vi "inst.Open.vi"(7 "unit ID in":u8=11, 8 "error in (no error)":errorcluster, 11 "VISA resource name":refnum<visa-resource-name>="COM4") -> (0 "error out":errorcluster, 3 "Modbus Master out":refnum<class "Modbus Master.lvclass">)   [LabVIEW 2018, in "MB Relay.lvlib"]
uses:
  MB Relay.lvlib
  <vilib>/NI/Modbus Library/API/Master/Modbus Master.lvclass
  <vilib>/NI/Modbus Library/API/Wrapper/Create Serial Master.vi
  <vilib>/NI/Modbus Library/API/Wrapper/API Main.lvlib
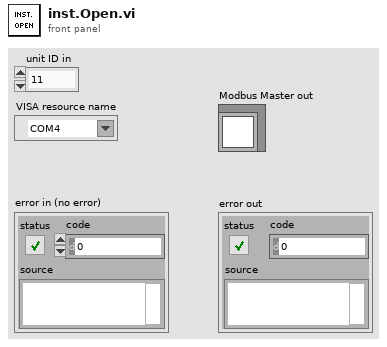
[diagram p1: front panel]
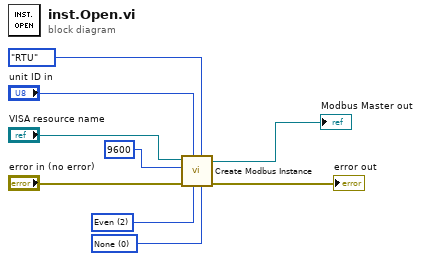
[diagram p0: block diagram]
diagram:
  w6 = u16 0 items=["None", "XON/XOFF", "RTS/CTS", "XON/XOFF & RTS/CTS", "DTR/DSR", "XON/XOFF & DTR/DSR"] ("flow control (none)")
  w5 = u16 2 items=["None", "Odd", "Even", "Mark", "Space"] ("parity (even)")
  n1 = call-poly <vilib>:"Create Modbus Instance.vi"("flow control (none)"=w6, "serial type"=enum16{"RTU", "ASCII"}."RTU", "parity (even)"=w5, "unit ID"="unit ID in", "error in"="error in (no error)", "baud rate"=u32 9600, "VISA resource name"="VISA resource name") -> ("error out"=→"error out":errorcluster, "serial master instance"=→"Modbus Master out":refnum<class "Modbus Master.lvclass">)  [unwired: 3 in]
